vi "WriteCalibrationFile.vi"(8 "error in (no error)":errorcluster, 10 "CalibrationState":T1, 11 "Path":path) -> (0 "error out":errorcluster)   [LabVIEW 2013]
panel:
  # "CalibrationDone"
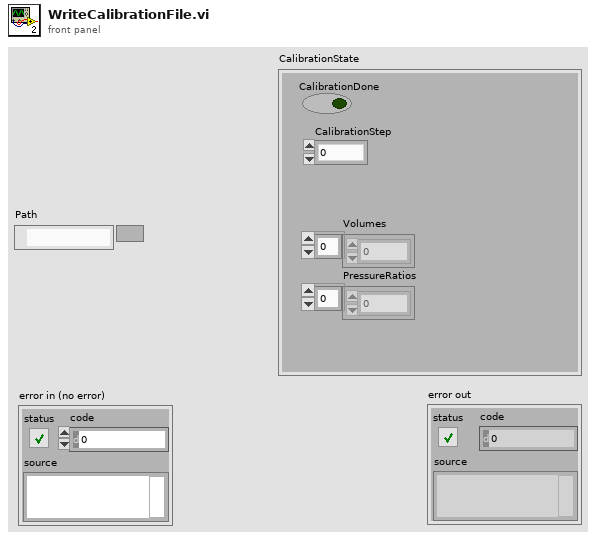
[diagram p1: front panel]
types:
  T1 = cluster{bool, "CalibrationStep":u32, "Volumes":dbl[], "PressureRatios":dbl[]}
  T2 = enum16{"open", "replace", "create", "open or create", "replace or create", "replace or create with confirmation"}
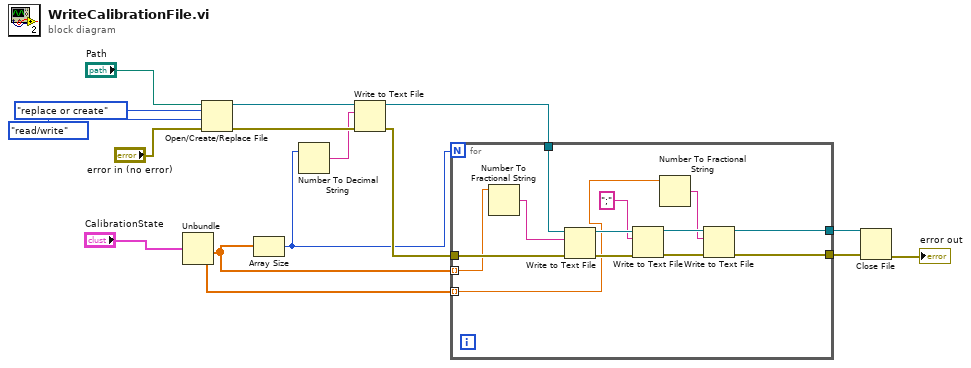
[diagram p0: block diagram]
diagram:
  n1 = Unbundle("CalibrationState") -> ("Volumes"=w2:dbl[], "PressureRatios"=w1:dbl[])  [unwired: 2 out]
  n2 = Open/Create/Replace File(file path (use dialog)="Path", error in="error in (no error)", operation (0:open)=T2."replace or create", access (0:read/write)=enum16{"read/write", "read-only", "write-only"}."read/write") -> (refnum out=w11:refnum<file>, error out=w10:errorcluster)  [unwired: 2 in, 1 out]
  n3 = Array Size(array=w2) -> (size(s)=w5:i32)
  n4 = Number To Decimal String(number=w5) -> (decimal integer string=w9:string)  [unwired: 1 in]
  n5 = Write to Text File(file (use dialog)=w11, text=w9, error in=w10) -> (refnum out=w3:refnum<file>, error out=w6:errorcluster)  [unwired: 1 in, 1 out]
  n6 = for {
    N: w5 -> [_]
    tunnel: [w29] -> w7
    tunnel: w6 -> [w28]
    tunnel: [w23] -> w4
    tunnel: w3 -> [w22]
    tunnel: w2 -> [w18] mode=indexing
    tunnel: w1 -> [w17] mode=indexing
    n7 = Number To Fractional String(number=w18) -> (F-format string=w20:string)  [unwired: 3 in]
    n8 = Write to Text File(file (use dialog)=w22, text=w20, error in=w28) -> (refnum out=w25:refnum<file>, error out=w27:errorcluster)  [unwired: 1 in, 1 out]
    n9 = Write to Text File(file (use dialog)=w25, text=";", error in=w27) -> (refnum out=w24:refnum<file>, error out=w26:errorcluster)  [unwired: 1 in, 1 out]
    n10 = Number To Fractional String(number=w17) -> (F-format string=w19:string)  [unwired: 3 in]
    n11 = Write to Text File(file (use dialog)=w24, text=w19, error in=w26) -> (refnum out=w23:refnum<file>, error out=w29:errorcluster)  [unwired: 1 in, 1 out]
  }
  n12 = Close File(refnum=w4, error in=w7) -> (error out=→"error out":errorcluster)  [unwired: 1 out]
